vi "Read Logger.vi"(8 "error in (no error)":errorcluster, 11 "Template Module in":refnum<class "Template Module.lvclass">) -> (0 "error out":errorcluster, 2 "Logger.lvclass":refnum<class "Logger.lvclass">, 3 "Template Module out":refnum<class "Template Module.lvclass">)   [LabVIEW 2018, in "Template Module.lvclass"]
uses:
  Template Module.lvclass
  Loggers/Logger/Logger.lvclass
  Template Module.lvclass/Template Module.ctl
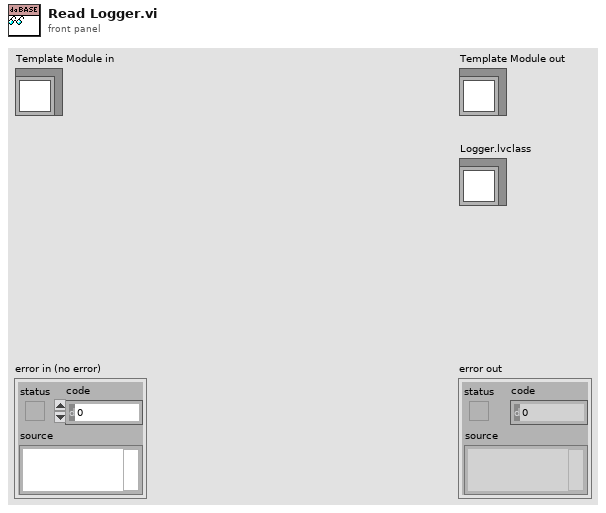
[diagram p1: front panel]
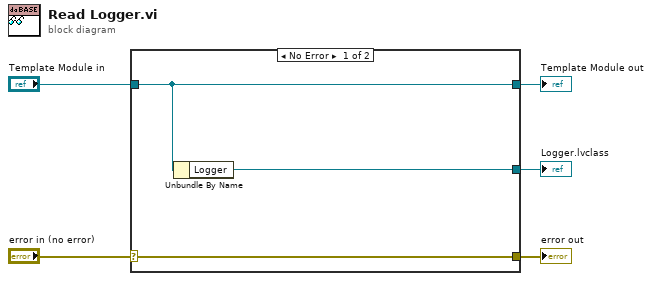
[diagram p0: block diagram]
diagram:
  n1 = case shown="No Error" "error in (no error)" {
    selector: "error in (no error)" -> [w8 w9]
    tunnel: [w8 w9] -> w4
    tunnel: [w7 w10] -> w2
    tunnel: "Template Module in" -> [w7 w10]
    tunnel: [w6 _] -> w1
    frame No Error {
      n2 = Unbundle By Name(w7) -> ("Logger"=w6:refnum<class "Logger.lvclass">)
    }
    frame Error {
    }
  }
  "error out" <- w4
  "Template Module out" <- w2
  "Logger.lvclass" <- w1
